vi "SubSystems.vi"(8 "error in":errorcluster) -> ()   [LabVIEW 2015]
doc: "This VI calls the various robot subsystems that will then run in parallel. New subSystems will automatlically script code to make the call."
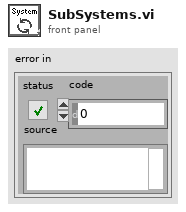
[diagram p1: front panel]
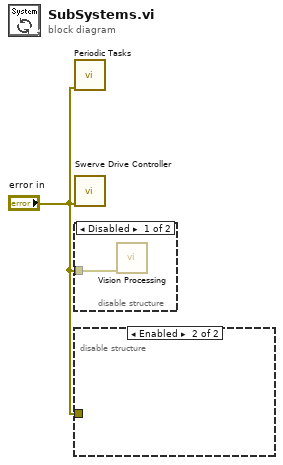
[diagram p0: block diagram]
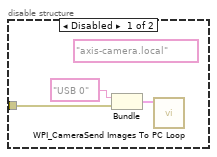
[diagram p3: hidden frame]
diagram:
  n1 = call "Periodic Tasks.vi"("error in"="error in") -> ()  [unwired: 1 in, 10 out]
  n2 = call "Swerve Drive Controller.vi"("error in"="error in") -> ()  [unwired: 11 in]
  n3 = disable-structure shown="Disabled" {
    disable-tunnel: "error in" -> [w2 _]
    frame Disabled {
      n4 = call "Vision Processing.vi"("error in (no error)"=w2) -> ()  [unwired: 7 in]
    }
    frame Enabled {
    }
  }
  n5 = disable-structure shown="Enabled" {
    disable-tunnel: "error in" -> [w3 _]
    frame Disabled {
      (unwired) "axis-camera.local" ("format string")
      n6 = Bundle("USB 0", "error in"=w3) -> (w4:cluster{string, "error in ":errorcluster})  [unwired: 1 in]
      n7 = call <vilib>:"WPI_CameraSend Images To PC Loop.vi"("CameraDevRef"=w4) -> ()  [unwired: 11 in]
    }
    frame Enabled {
    }
  }
